vi "Update AOs Values.vi"(8 "error in":errorcluster, 9 "Remote UDP Listening Port":u16, 10 "Remote IP":string, 11 "AIs Values":sgl[](array[numeric])) -> (0 "error out":errorcluster)   [LabVIEW 2021, in "RT Interpreter Manager.lvlib"]
uses:
  RT Interpreter Manager.lvlib
  Libraries/UDP Comms/UDP Message--cluster.ctl
  Libraries/UDP Comms/UDP Comms.lvlib
panel:
  out "AOs Values":sgl[](array[numeric])
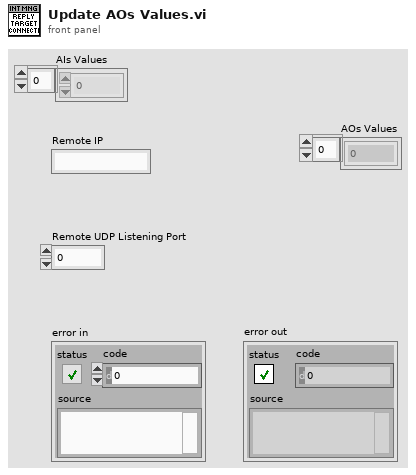
[diagram p1: front panel]
types:
  T1 = typedef "UDP Comms.lvlib/UDP Message--cluster.ctl" = cluster{"Command":string, "Data":variant}
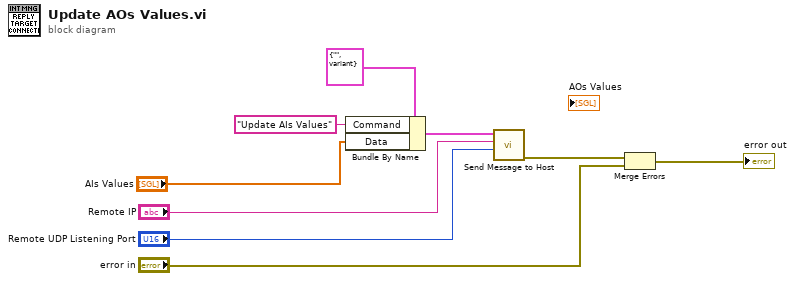
[diagram p0: block diagram]
diagram:
  n1 = Bundle By Name(cluster=T1 {"Command"="", "Data"=variant} ("UDP Message"), "Command"="Update AIs Values", "Data"="AIs Values") -> (w8:T1)
  n2 = call "Send Message to Host.vi"("Remote UDP Listening Port"="Remote UDP Listening Port", "Remote IP"="Remote IP", "UDP Message"=w8) -> ("error out"=w4:errorcluster)  [unwired: 8 in]
  n3 = Merge Errors(w4, "error in") -> (→"error out":errorcluster)
